vi "Acquire.vi"(8 "error in (no error)":errorcluster, 9 "Data Queue":refnum<queue>, 10 "Data Notifier":refnum<notifier>, 11 "Hardware Configuration In":T2) -> (0 "error out":errorcluster, 3 "Hardware Configuration Out":T2)   [LabVIEW 2022 SP3, in "Acquisition.lvlib"]
doc: "Perform the acquisition. Replace the contents of this diagram with calls to acquisition hardware."
uses:
  Acquisition.lvlib
  Logging/QueuedLoggedData.ctl
  FFT-Data.ctl
  FiniteMeasurement-DAQmx/controls/Hardware Configuration.ctl
  WhiteNoise.ctl
  <vilib>/Analysis/3filter.llb/Filter Passband Type.ctl
  <vilib>/DAQmx/read.llb/DAQmx Read (Analog 1D Wfm NChan NSamp).vi
  <vilib>/DAQmx/miscellaneous.llb/DAQmx Fill In Error Info.vi
  <vilib>/Analysis/3filter.llb/Butterworth Filter (DBL).vi
  <resource>/objmgr/daqmx.rc
  <vilib>/Analysis/NI_AALBase.lvlib
panel:
  in  "Filter":cluster{"Upper Cutoff":T1, "Lower Cutoff":T1}={"Upper Cutoff"=350.0, "Lower Cutoff"=350.0}
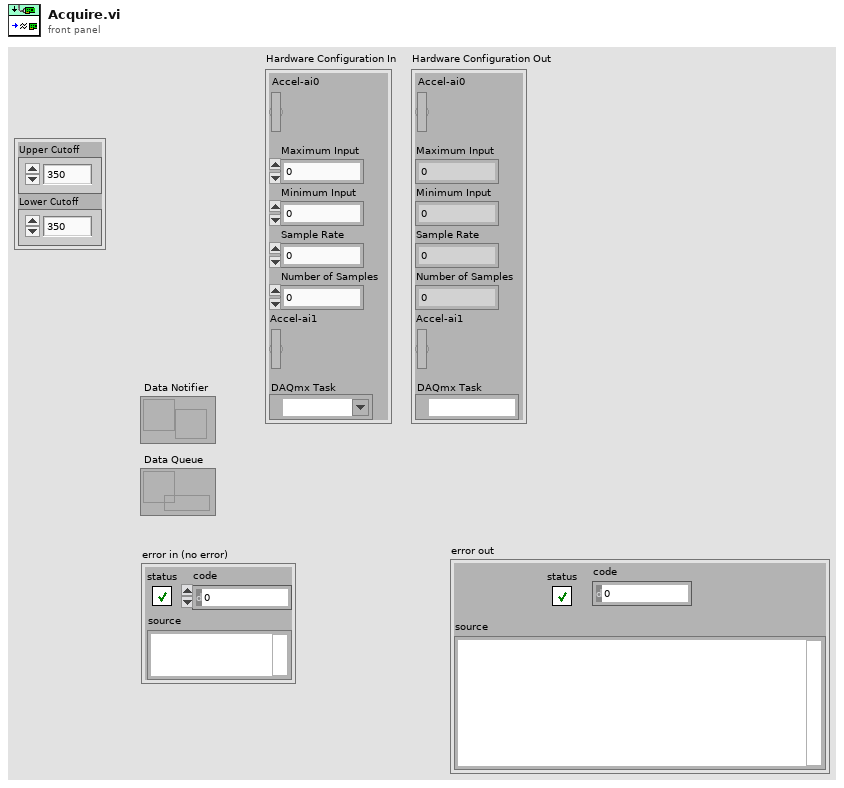
[diagram p1: front panel]
types:
  T1 = typedef "WhiteNoise.ctl" = dbl
  T2 = typedef "Acquisition.lvlib/Hardware Configuration.ctl" = cluster{"Accel-ai0":bool, "Maximum Input":dbl, "Minimum Input":dbl, "Sample Rate":dbl, "Number of Samples":i32, "Accel-ai1":bool, "DAQmx Task":refnum<k21>}
  T3 = typedef "QueuedLoggedData.ctl" = cluster{"RawData":waveform(dbl)[], "FFT ":T4[]}
  T4 = typedef "FFT-Data.ctl" = cluster{"FFT-Mag":cluster{"t0":dbl, "dt":dbl, "Y":dbl[]}, "FFT-Phase":cluster{"t0":dbl, "dt":dbl, "Y":dbl[]}}
  T5 = typedef "NI_AALBase.lvlib/Filter Passband Type.ctl" = enum32{"Lowpass", "Highpass", "Bandpass", "Bandstop"}
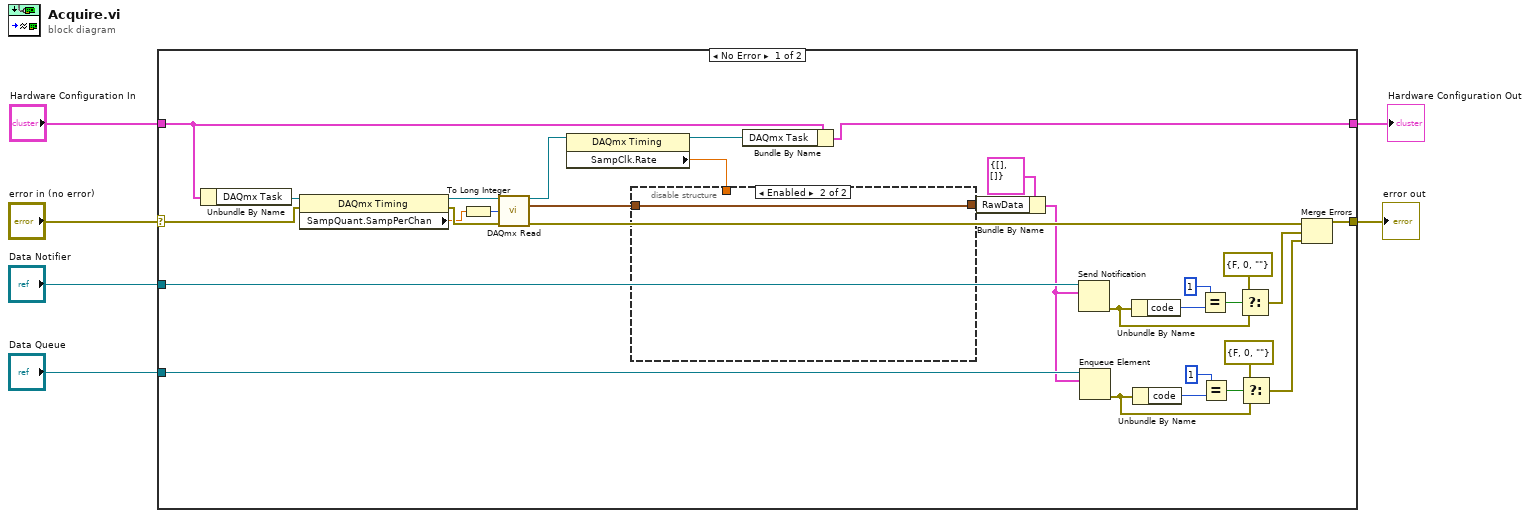
[diagram p0: block diagram]
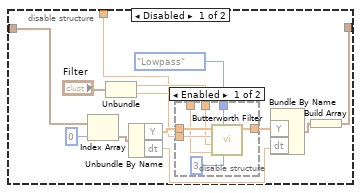
[diagram p2: hidden frame]
diagram:
  n1 = case shown="No Error" "error in (no error)" {
    selector: "error in (no error)" -> [w34 w60]
    tunnel: [w37 w60] -> w5
    tunnel: "Hardware Configuration In" -> [w32 w61]
    tunnel: [w33 w61] -> w1
    tunnel: "Data Notifier" -> [w36 _]
    tunnel: "Data Queue" -> [w35 _]
    frame No Error {
      n2 = Unbundle By Name(w32) -> ("DAQmx Task"=w18:refnum<k21>)
      n3 = property class="DAQmx Timing"(reference=w18, error in=w34) -> (reference out=w17:refnum<k21>, error out=w16:errorcluster, "SampQuant.SampPerChan"=w15:dbl)
      n4 = To Long Integer(number=w15) -> (32bit integer=w14:i32)
      n5 = call-poly <vilib>:"DAQmx Read.vi"("task/channels in"=w17, "number of samples per channel"=w14, "error in"=w16) -> ("task out"=w13:refnum<k21>, "data"=w8:waveform(dbl)[], "error out"=w19:errorcluster)  [unwired: 10 in]
      n6 = property class="DAQmx Timing"(reference=w13) -> (reference out=w10:refnum<k21>, "SampClk.Rate"=w9:dbl)  [unwired: 1 in, 1 out]
      n7 = disable-structure shown="Enabled" {
        disable-tunnel: w9 -> [w43 _]
        disable-tunnel: w8 -> [w41 w59]
        disable-tunnel: [w39 w59] -> w7
        frame Disabled {
          n8 = Index Array(array=w41, index=0) -> (element=w45:waveform(dbl))
          n9 = Unbundle("Filter") -> ("Upper Cutoff"=w49:T1, "Lower Cutoff"=w50:T1)
          n10 = Unbundle By Name(w45) -> ("Y"=w47:dbl[], "dt"=w38:dbl)
          n11 = disable-structure shown="Enabled" {
            disable-tunnel: Filter_Passband_Type."Lowpass" ("filter type") -> [w57 _]
            disable-tunnel: w47 -> [w56 w58]
            disable-tunnel: w43 -> [w55 _]
            disable-tunnel: w50 -> [w54 _]
            disable-tunnel: w49 -> [w53 _]
            disable-tunnel: [w51 w58] -> w42
            frame Enabled {
              n12 = call-poly <vilib>:"Butterworth Filter.vi"("order"=3, "filter type"=w57, "low cutoff freq: fl"=w54, "high cutoff freq: fh"=w53, "sampling freq: fs"=w55, "X"=w56) -> ("Filtered X"=w51:dbl[])  [unwired: 2 in, 1 out]
            }
            frame Disabled {
            }
          }
          n13 = Bundle By Name("Y"=w42, "dt"=w38) -> (w40:waveform(dbl))  [unwired: 1 in]
          n14 = Build Array(w40) -> (w39:waveform(dbl)[])
        }
        frame Enabled {
        }
      }
      n15 = Bundle By Name(cluster=w32, "DAQmx Task"=w10) -> (w33:T2)
      n16 = Bundle By Name(cluster=T3 {"RawData"=[], "FFT "=[]} ("Cluster"), "RawData"=w7) -> (w11:T3)
      n17 = Send Notification(notification=w11, notifier=w36) -> (error out=w28:errorcluster)  [unwired: 1 in, 1 out]
      n18 = Enqueue Element(queue=w35, element=w11) -> (error out=w24:errorcluster)  [unwired: 2 in, 2 out]
      n19 = Unbundle By Name(w28) -> ("code"=w31:i32)
      n20 = Unbundle By Name(w24) -> ("code"=w21:i32)
      n21 = Equal?(x=1, y=w31) -> (x = y?=w29:bool)
      n22 = Equal?(x=1, y=w21) -> (x = y?=w23:bool)
      n23 = Select(t=errorcluster {"status"=FALSE, "code"=0, "source"=""} ("error constant"), s=w29, f=w28) -> (s? t:f=w27:errorcluster)
      n24 = Select(t=errorcluster {"status"=FALSE, "code"=0, "source"=""} ("error constant"), s=w23, f=w24) -> (s? t:f=w20:errorcluster)
      n25 = Merge Errors(w19, w27, w20) -> (w37:errorcluster)
    }
    frame Error {
    }
  }
  "error out" <- w5
  "Hardware Configuration Out" <- w1
